vi "DB Close.vi"(8 "error in":errorcluster, 11 "Database in":refnum<class "Database.lvclass">) -> (0 "error out":errorcluster, 3 "Database out":refnum<class "Database.lvclass">)   [LabVIEW 2023, in "HardwareAbstractionLayer_LVOOP.lvlib" / "Database.lvclass"]
doc: "This VI is Database Close Reference"
uses:
  Database.lvclass
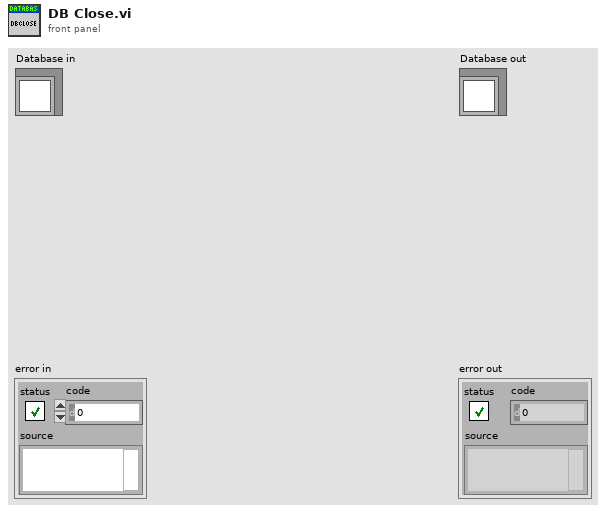
[diagram p1: front panel]
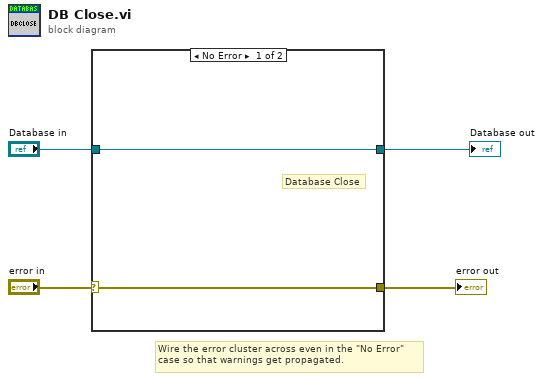
[diagram p0: block diagram]
diagram:
  # "Wire the error cluster across even in the \"No Error\"\ncase so that warnings get propagated."
  n1 = case shown="No Error" "error in" {
    selector: "error in" -> [w5 w8]
    tunnel: [w5 w8] -> w3
    tunnel: [w6 w7] -> w1
    tunnel: "Database in" -> [w6 w7]
    frame No Error {
      # "Database Close"
    }
    frame Error {
    }
  }
  "error out" <- w3
  "Database out" <- w1
